vi "AK Timeout.vi"(6 "Aktionen":T1, 8 "Fehler":errorcluster caption="Fehler (Eingang, kein Fehler)", 10 "Zeitstempel":timestamp) -> (2 "Zeitstempel":timestamp, 4 "Aktionen":T1)   [LabVIEW 2020, in "FT-IR.lvlib" / "AK-Interface.lvlib"]
uses:
  AK-Interface.lvlib
  Aktionen AK.ctl
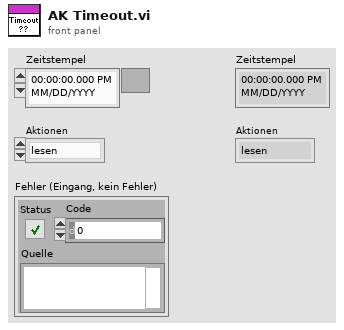
[diagram p1: front panel]
types:
  T1 = typedef "FT-IR.lvlib/AK-Interface.lvlib/Aktionen AK.ctl" = enum16{"lesen", "initialisieren", "beenden", "AK Komm"}
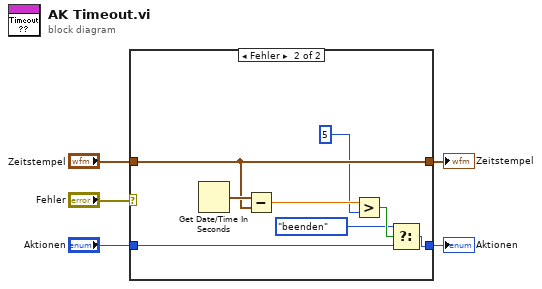
[diagram p0: block diagram]
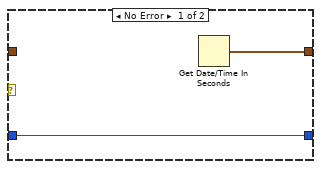
[diagram p2: hidden frame]
diagram:
  n1 = case shown="Fehler" "Fehler" {
    tunnel: [w7 w14] -> w1
    tunnel: "Zeitstempel" -> [_ w14]
    tunnel: "Aktionen" -> [w6 w11]
    tunnel: [w6 w9] -> w5
    frame No Error {
      n2 = Get Date/Time In Seconds() -> (seconds since 1Jan1904=w7:timestamp)
    }
    frame Error {
      n3 = Get Date/Time In Seconds() -> (seconds since 1Jan1904=w15:timestamp)
      n4 = Subtract(x=w15, y=w14) -> (x-y=w13:dbl)
      n5 = Greater?(x=w13, y=u16 5 ("Timeout")) -> (0:w12:bool)
      n6 = Select(t=Aktionen_AK."beenden" ("Aktionen"), s=w12, f=w11) -> (s? t:f=w9:T1)
    }
  }
  "Aktionen" <- w5
  "Zeitstempel" <- w1
